vi "PKG_IMC_GetParam16.vi"(7 "axis":i32, 9 "data":i16, 10 "paramloc":i16, 11 "Handle":u32) -> (1 "data out":i16, 2 "function return":i32, 3 "Handle out":u32)   [LabVIEW 2011, in "IMC_Pkg4xxx.lvlib"]
doc: "PKG_IMC_GetParam16(IMC_HANDLE Handle, short paramloc, short* data, int axis);"
uses:
  IMC_Pkg4xxx.lvlib
  IMC_Pkg4xxx.dll
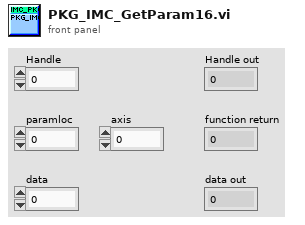
[diagram p1: front panel]
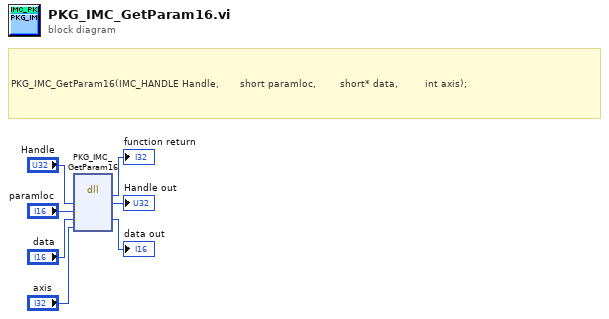
[diagram p0: block diagram]
diagram:
  # "PKG_IMC_GetParam16(IMC_HANDLE Handle, \t\t\t\t\t\tshort paramloc, \t\t\t\t\t\t\tshort* data, \t\t\t\t\t\t\t\tint axis);"
  n1 = dll-call lib="PTH1mabs F光盘刻录\niMC MotionIMCNet_V4.0IMCAppincLabviewIMC_PKG4xxxIMC_PKG4xxx\nIMC_Pkg4xxx.*" fn="PKG_IMC_GetParam16"("Handle"="Handle", "paramloc"="paramloc", "data"="data", "axis"="axis") -> (→"function return":i32, "Handle"=→"Handle out":u32, "data"=→"data out":i16)  [unwired: 5 in, 2 out]
